vi "TagDB Example.vi"() -> ()   [LabVIEW 2017]
uses:
  cff7abee-2af5-461c-929f-3f62dc38e682.vi
  ff38bd82-3f9e-4f53-9d41-be54fc07b73c.vi
  dcf35176-e820-41a0-ad54-6b9ac1d48946.vi
  4329e122-b20c-4910-b184-414f52bef2b4.vi
  0432307d-c668-4f11-a04e-5d0627652fdc.vi
  8b2616c1-f426-4650-a165-5f39781f1ade.vi
  971914ca-3885-4006-86c3-c9477108d6ff.vi
  TagDB/_Support/DataAccess/data-Write.vi
  TagDB/_Support/Error/_[error50000]Invalid DB REF.vi
  TagDB/_Support/DataAccess/TagDB Ref to DVR.vi
  TagDB/_Support/DataAccess/_NameCacher.vi
  TagDB/_Support/Error/_[error50002]Invalid DataType.vi
  TagDB/_Support/URL/TRIM-BOTH-SPACE.vi
  TagDB/_Support/DataAccess/_datatypeChecker.vi
  <vilib>/Utility/Data Type/Get Type Information.vi
  TagDB/_Support/Error/_Build Error Cluster.vi
  TagDB/TagDB.lvlib
panel:
  out "Not Predef Tag":string
  out "value 2":variant
  out "DataItemFlag":timestamp
  out "DataChangeFlag":timestamp
  in  "value":string="test send message"
  out "String":string
  in  "stop":bool
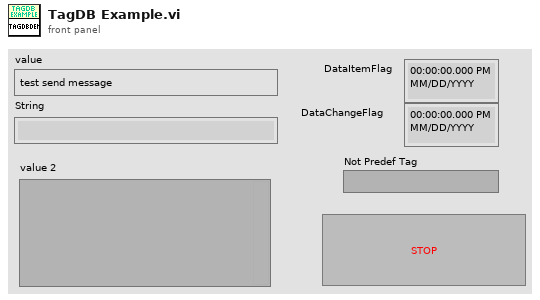
[diagram p1: front panel]
types:
  T1 = cluster{"number":i32, "boolean":bool, "abcdef":cluster{"number":i32, "boolean":bool}}
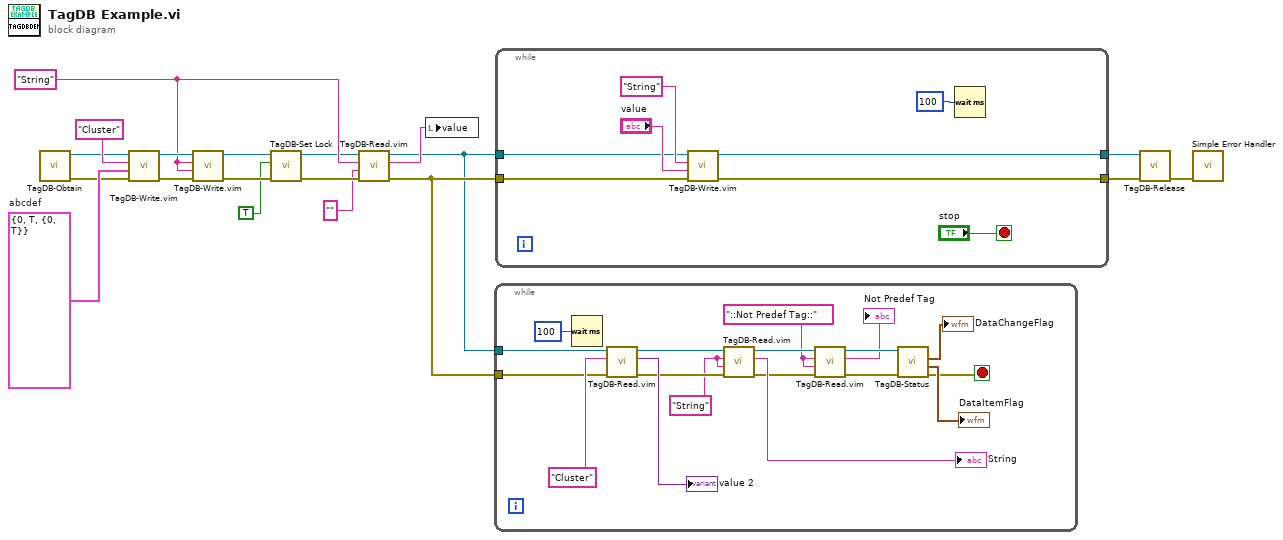
[diagram p0: block diagram]
diagram:
  w11 = T1 {"number"=0, "boolean"=TRUE, "abcdef"={"number"=0, "boolean"=TRUE}}  # abcdef
  w8 = "String" ("String")
  n1 = call "TagDB-Obtain.vi"() -> ("error out"=w10:errorcluster, "TagDB"=w2:refnum<k1>)  [unwired: 5 in, 1 out]
  n2 = call "TagDB-Write.vim"("error in (no error)"=w10, "Value"=w11, "tag"="Cluster" ("name"), "TagDB"=w2) -> ("error out"=w13:errorcluster, "TagDB(dup)"=w14:refnum<k1>)  [unwired: 5 in, 1 out]
  n3 = call "TagDB-Write.vim"("error in (no error)"=w13, "Value"=w8, "tag"=w8, "TagDB"=w14) -> ("error out"=w6:errorcluster, "TagDB(dup)"=w15:refnum<k1>)  [unwired: 5 in, 1 out]
  n4 = call "TagDB-Set Lock.vi"("error in (no error)"=w6, "Lock?(T)"=TRUE ("Lock?"), "TagDB"=w15) -> ("error out"=w5:errorcluster, "TagDB(dup)"=w7:refnum<k1>)  [unwired: 7 in]
  n5 = call "TagDB-Read.vim"("error in (no error)"=w5, "Type(empty to read as variant)"="" ("Type"), "name"=w8, "TagDB"=w7) -> ("error out"=w17:errorcluster, "Value"=w16:string, "TagDB(dup)"=w1:refnum<k1>)  [unwired: 2 in, 3 out]
  n6 = local write "value"(w16) -> ()
  n7 = while {
    tunnel: w1 -> [w30]
    tunnel: w17 -> [w28]
    stop <- w31 stop-if-true
    w20 = "::Not Predef Tag::" ("name")
    w26 = "String" ("name")
    n8 = Wait (ms)(milliseconds to wait=u32 100) -> ()  [unwired: 1 out]
    n9 = call "TagDB-Read.vim"("error in (no error)"=w28, "name"="Cluster", "TagDB"=w30) -> ("error out"=w27:errorcluster, "Value"=→"value 2":variant, "TagDB(dup)"=w29:refnum<k1>)  [unwired: 3 in, 3 out]
    n10 = call "TagDB-Read.vim"("error in (no error)"=w27, "Type(empty to read as variant)"=w26, "name"=w26, "TagDB"=w29) -> ("error out"=w24:errorcluster, "Value"=→"String":string, "TagDB(dup)"=w25:refnum<k1>)  [unwired: 2 in, 3 out]
    n11 = call "TagDB-Read.vim"("error in (no error)"=w24, "Type(empty to read as variant)"=w20, "name"=w20, "TagDB"=w25) -> ("error out"=w23:errorcluster, "Value"=→"Not Predef Tag":string, "TagDB(dup)"=w22:refnum<k1>)  [unwired: 2 in, 3 out]
    n12 = call "TagDB-Status.vi"("error in (no error)"=w23, "DB Ref"=w22) -> ("error out"=w31:errorcluster, "Item Change Timestamp"=→"DataItemFlag":timestamp, "Global Change Timestamp"=→"DataChangeFlag":timestamp)  [unwired: 4 in, 3 out]
  }
  n13 = while {
    tunnel: w1 -> [w40]
    tunnel: w17 -> [w41]
    tunnel: [w39] -> w9
    tunnel: [w42] -> w18
    stop <- "stop" stop-if-true
    n14 = call "TagDB-Write.vim"("error in (no error)"=w41, "Value"="value", "tag"="String" ("name"), "TagDB"=w40) -> ("error out"=w39:errorcluster, "TagDB(dup)"=w42:refnum<k1>)  [unwired: 5 in, 1 out]
    n15 = Wait (ms)(milliseconds to wait=u32 100) -> ()  [unwired: 1 out]
  }
  n16 = call "TagDB-Release.vi"("error in (no error)"=w9, "TagDB"=w18) -> ("error out"=w19:errorcluster)  [unwired: 9 in]
  n17 = call <vilib>:"Simple Error Handler.vi"("error in (no error)"=w19) -> ()  [unwired: 4 in, 5 out]
